vi "Unicode Encode.vi"(7 "个数":i32, 11 "字符串":string) -> (3 "数组":u8[](array[numeric]) format="%02x")   [LabVIEW 2016, in "DGUS.lvlib" / "DGUS.lvclass"]
uses:
  DGUS.lvclass
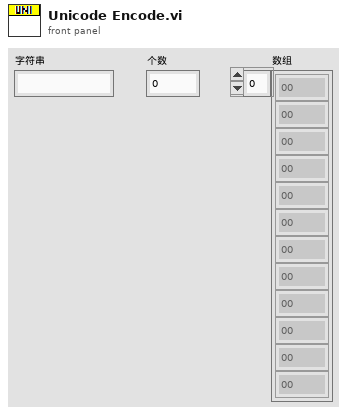
[diagram p1: front panel]
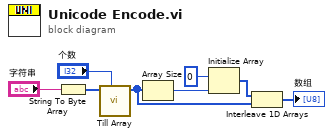
[diagram p0: block diagram]
diagram:
  n1 = String To Byte Array(string="字符串") -> (unsigned byte array=w4:u8[])
  n2 = call "Till Array.vi"("字节个数"="个数", "input"=w4) -> ("output"=w2:u8[])  [unwired: 9 in]
  n3 = Array Size(array=w2) -> (size(s)=w7:i32)
  n4 = Initialize Array(u8 0, w7) -> (w5:u8[])
  n5 = Interleave 1D Arrays(w5, w2) -> (→"数组":u8[])
